vi "Principal.vi"() -> ()   [LabVIEW 2014]
panel:
  in  "Cluster":T1
  in  "confEnsaioButton 2":bool
  out "ledVibracao":bool caption="Vibração"
  out "ledCarga":bool caption="Célula"
  out "ledRotacao":bool caption="Rotação"
  out "ledTermoparRef":bool caption="Termopar Ref"
  out "ledTermoparB":bool caption="Termopar B"
  out "ledTermoparA":bool caption="Termopar A"
  in  "pathToFile":path
  in  "Boolean 2":bool
  in  "Boolean":bool
  in  "stopButton":bool
  in  "confEnsaioButton":bool
  in  "calibraButton":bool
  in  "sobreButton":bool
  in  "startButton":bool
  out "Freio":bool
  out "Motor":bool
  in  "Ring":u16(ring) items=["Vi 3", "Vi 2", "Vi 1"]
  # "-"
  # "001"
  # "999"
  # "Bancada de Frenagem - Ensaio"
  # "Sensores"
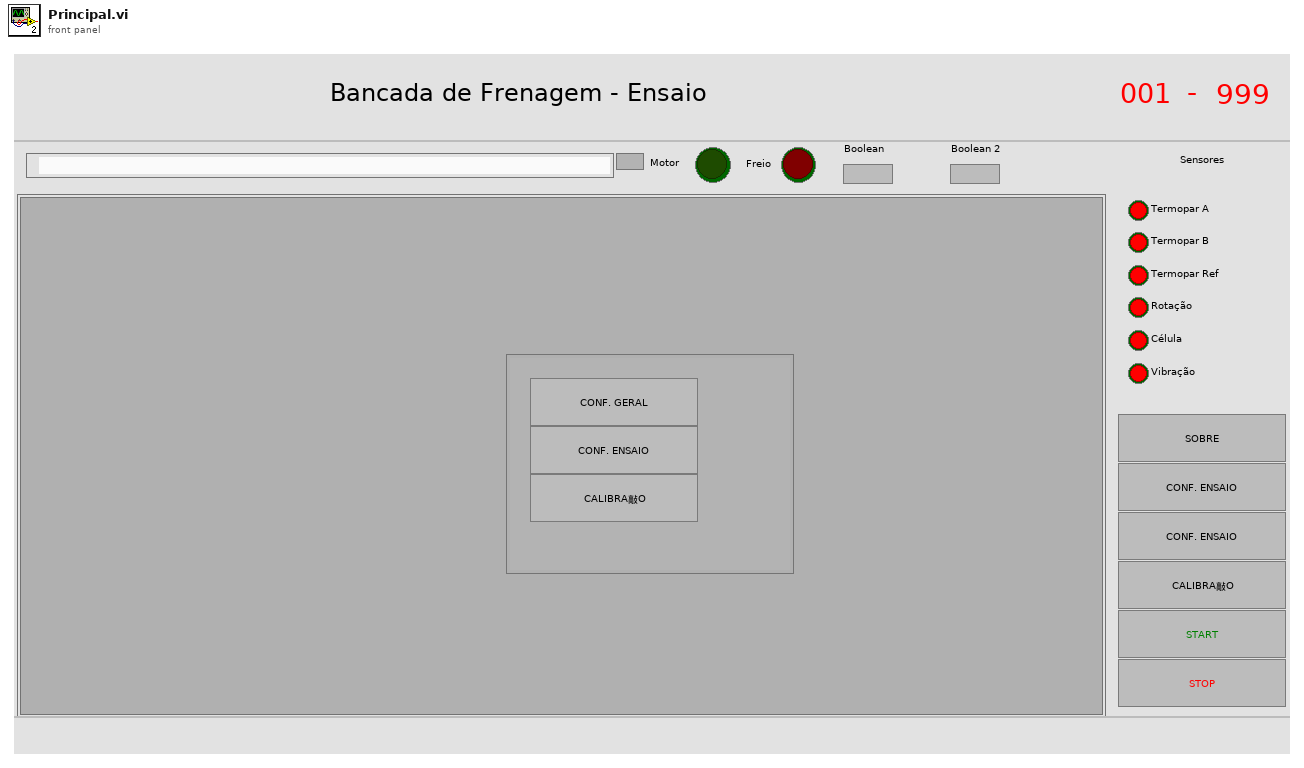
[diagram p1: front panel]
types:
  T1 = cluster{"confGeralButton":bool, "confEnsaioButton":bool, "calibraButton":bool}
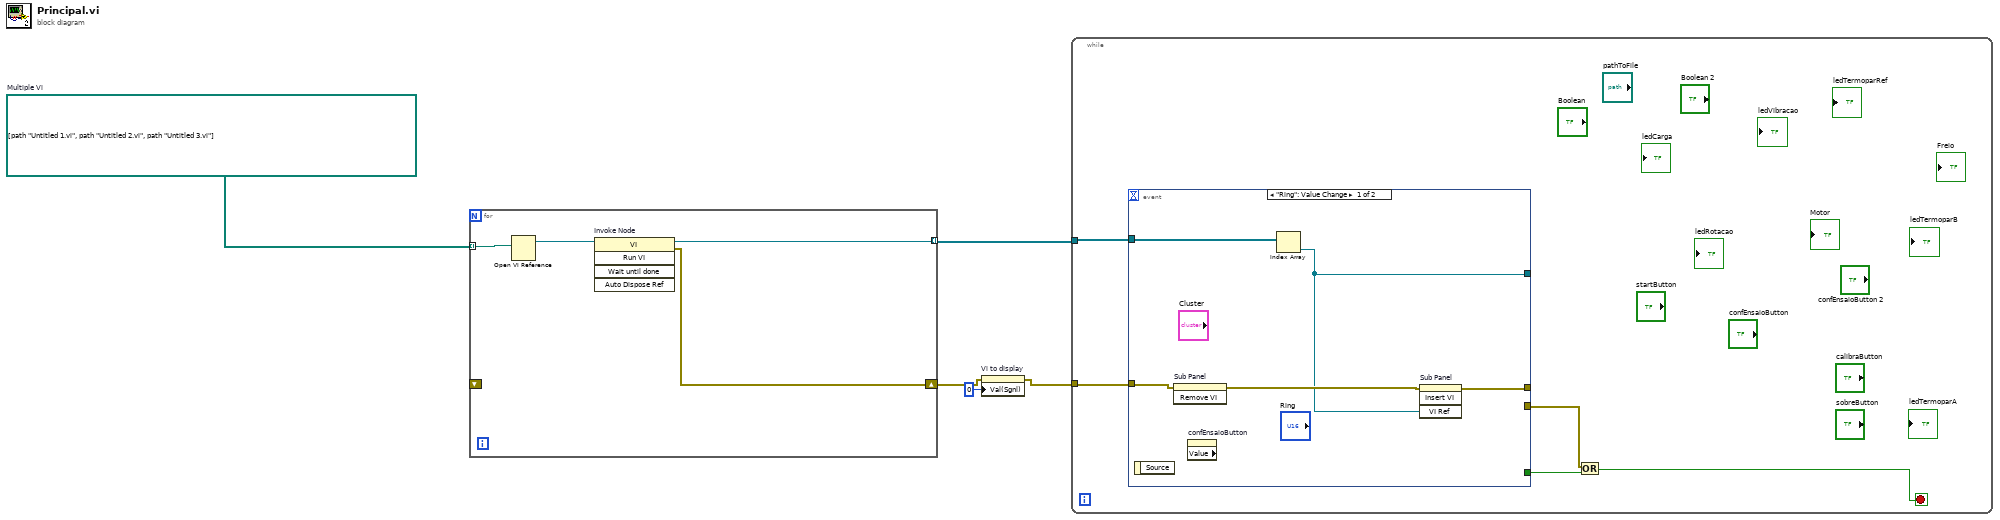
[diagram p0: block diagram]
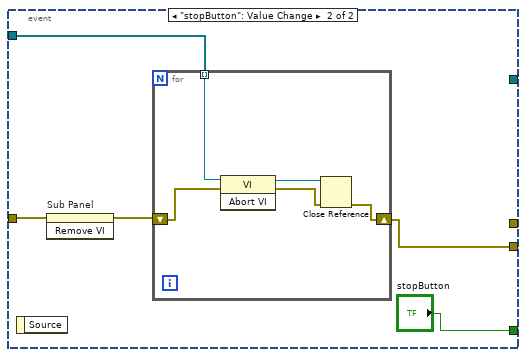
[diagram p2: hidden frame]
diagram:
  w5 = path[] [path "Untitled 1.vi", path "Untitled 2.vi", path "Untitled 3.vi"]  # Multiple Vi
  n1 = for {
    tunnel: w5 -> [w9] mode=indexing
    shift-right: [w7] -> w3
    shift-left: _ -> [_]
    tunnel: [w6] -> w4 mode=indexing
    n2 = Open VI Reference(vi path=w9) -> (vi reference=w8:refnum<vi>)  [unwired: 5 in, 1 out]
    n3 = invoke on="Invoke Node" class="VI" method="Run VI"(reference=w8) -> (reference out=w6:refnum<vi>, error out=w7:errorcluster)  [unwired: 4 in, 3 out]
  }
  n4 = property on="Vi to display" class="Ring (strict)"(error in=w3, "Val(Sgnl)"=u16 0 ("Value (Signaling)")) -> (error out=w2:errorcluster)  [unwired: 1 in, 1 out]
  n5 = while {
    tunnel: w4 -> [w13]
    tunnel: w2 -> [w14]
    stop <- w10 stop-if-true
    n6 = event shown="[0] \"Ring\": Value Change" {
      selector: _ -> [_ _]
      dyn-events: _ -> [_ _]
      timeout: _ -> [_ _]
      tunnel: w14 -> [w19 w21]
      tunnel: w13 -> [w17 w24]
      tunnel: [w16 _] -> _
      tunnel: [w15 _] -> _
      tunnel: [_ w20] -> w12
      tunnel: [_ "stopButton"] -> w11
      event "Ring": Value Change {
        n7 = event-data() -> ()  [unwired: 1 in, 1 out]
        n8 = invoke on="Sub Panel" class="SubPnl" method="Remove VI"(error in=w19) -> (error out=w18:errorcluster)  [unwired: 2 in, 2 out]
        n9 = property on="confEnsaioButton" class="Bool" props=["Value"]() -> ()  [unwired: 2 in, 3 out]
        n10 = Index Array(array=w17) -> (element=w15:refnum<vi>)  [unwired: 1 in]
        n11 = invoke on="Sub Panel" class="SubPnl" method="Insert VI"(error in=w18, "VI Ref"=w15) -> (error out=w16:errorcluster)  [unwired: 2 in, 3 out]
      }
      event "stopButton": Value Change {
        n12 = event-data() -> ()  [unwired: 1 in, 1 out]
        n13 = invoke on="Sub Panel" class="SubPnl" method="Remove VI"(error in=w21) -> (error out=w22:errorcluster)  [unwired: 2 in, 2 out]
        n14 = for {
          tunnel: w24 -> [w29] mode=indexing
          shift-right: [w25] -> w20
          shift-left: w22 -> [w26]
          n15 = invoke class="VI" method="Abort VI"(reference=w29, error in=w26) -> (reference out=w28:refnum<vi>, error out=w27:errorcluster)  [unwired: 1 in, 1 out]
          n16 = Close Reference(reference=w28, error in (no error)=w27) -> (error out=w25:errorcluster)
        }
      }
    }
    n17 = Or(x=w12, y=w11) -> (x .or. y?=w10:bool)
  }
